vi "05-RandomNumbers2.vi"() -> ()   [LabVIEW 2019]
panel:
  out "Loop Count":dbl
  out "Random Number":dbl
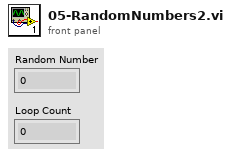
[diagram p1: front panel]
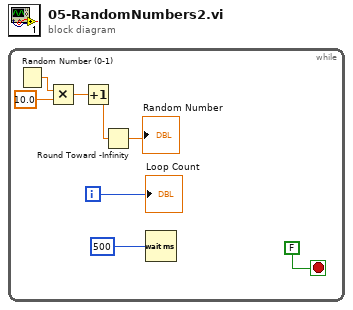
[diagram p0: block diagram]
diagram:
  n1 = while {
    i -> [w8]
    stop <- FALSE stop-if-true
    n2 = Random Number (0-1)() -> (number: 0 to 1=w5:dbl)
    n3 = Multiply(x=w5, y=10.0) -> (x*y=w3:dbl)
    n4 = Increment(x=w3) -> (x+1=w1:dbl)
    n5 = Round Toward -Infinity(1:w1) -> (0:→"Random Number":dbl)
    n6 = Wait (ms)(milliseconds to wait=u32 500) -> ()  [unwired: 1 out]
    "Loop Count" <- w8
  }
